vi "leakage protection.vi"(7 "matrix size":i32, 10 "index in":i32) -> (3 "index out":i32)   [LabVIEW 2017]
doc: "本VI就是用于检查控件索引值是否超过数组下标最大值的。\n如果超过，则强制转换回来。"
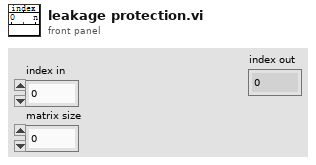
[diagram p1: front panel]
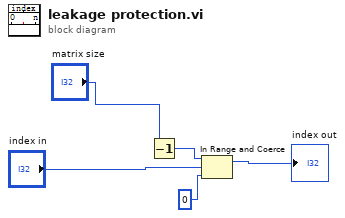
[diagram p0: block diagram]
diagram:
  n1 = Decrement(x="matrix size") -> (x-1=w4:i32)
  n2 = In Range and Coerce(upper limit=w4, x="index in", lower limit=0 ("下限")) -> (coerced(x)=→"index out":i32)  [unwired: 1 out]
